vi "Write Current Actual.vi"   [LabVIEW 2023, in "Power Supply.lvclass"]
uses:
  Power Supply.lvclass
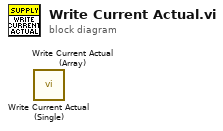
[diagram p0: block diagram]
diagram:
  n1 = call "Write Current Actual (Single).vi"() -> ()  [unwired: 10 in, 2 out]
  n2 = call "Write Current Actual (Array).vi"() -> ()  [unwired: 10 in, 2 out]
